vi "Query Multi Eval Meas Trigger Source Catalog.vi"(8 "error in (no error)":errorcluster, 10 "Instance (1)":i32=1, 11 "VISA resource name":refnum<visa-resource-name>) -> (0 "error out":errorcluster, 2 "Catalog":string[](array[string]), 3 "VISA resource name out":refnum<visa-resource-name>)   [LabVIEW 2020, in "Rohde&Schwarz CMP LR WPAN Measurement.lvlib"]
doc: "Lists all trigger source values that can be set using TRIGger:WPAN:MEAS<i>:MEValuation:SOURce.\n\nAttribute:\n-\n\nRemote-control command:\nTRIGger:WPAN:MEAS<i>:MEValuation:CATalog:SOURce?"
uses:
  <instrlib>/Rohde&Schwarz CMP LR WPAN Measurement/Rohde&Schwarz CMP LR WPAN Measurement.lvlib
  <instrlib>/Rohde&Schwarz CMP LR WPAN Measurement/Private/rsidr_core.llb/rsidr_core.lvlib
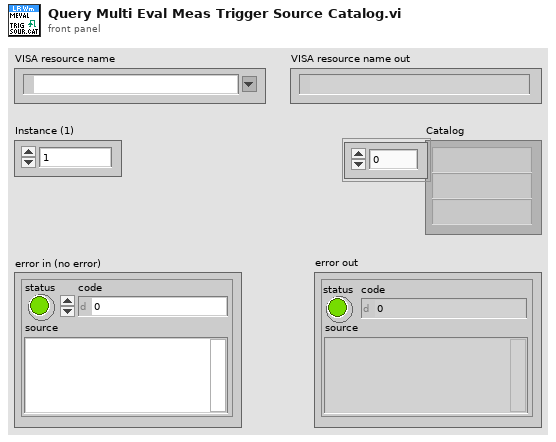
[diagram p1: front panel]
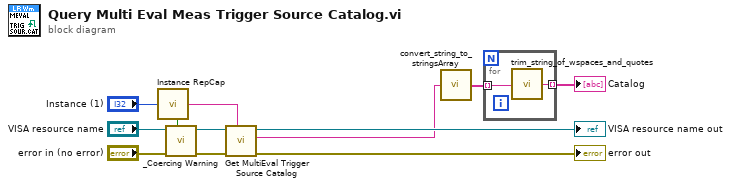
[diagram p0: block diagram]
diagram:
  n1 = call <instrlib>:"Instance RepCap.vi"("Instance In"="Instance (1)") -> ("In Range?"=w11:bool, "RepCap Identifier Out"=w12:string)  [unwired: 1 in]
  n2 = call <instrlib>:"_Coercing Warning.vi"("In Range?"=w11, "error in (no error)"="error in (no error)", "VISA resource name"="VISA resource name") -> ("error out"=w6:errorcluster, "VISA resource name out"=w5:refnum<visa-resource-name>)  [unwired: 7 in]
  n3 = call "Get MultiEval Trigger Source Catalog"("Repeated Capabilities"=w12, "error in (no error)"=w6, "instrument handle"=w5) -> ("error out"=→"error out":errorcluster, "MultiEval Trigger Source Catalog"=w1:string, "instrument handle out"=→"VISA resource name out":refnum<visa-resource-name>)  [unwired: 6 in]
  n4 = call <instrlib>:"convert_string_to_stringsArray.vi"("String in"=w1) -> ("string array out"=w10:string[])  [unwired: 3 in, 1 out]
  n5 = for {
    tunnel: w10 -> [w13] mode=indexing
    tunnel: [w14] -> w9 mode=indexing
    n6 = call <instrlib>:"trim_string_of_wspaces_and_quotes.vi"("String in"=w13) -> ("String out"=w14:string)  [unwired: 4 in]
  }
  "Catalog" <- w9
